vi "JoyToFps.vi"(8 "FpsInput Right":dbl, 9 "FpsInput Left":dbl, 11 "JoystickInput":dbl) -> (0 "Joystick Right":dbl, 1 "Joystick Left":dbl, 3 "Fps":dbl)   [LabVIEW 2020]
doc: "Converts JoystickInput to Fps on top and Fps to joystick on bottom"
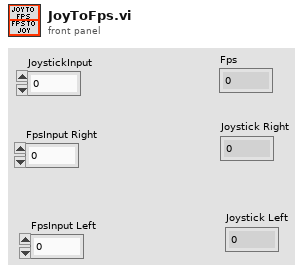
[diagram p1: front panel]
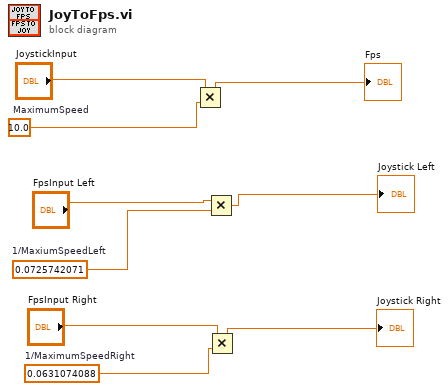
[diagram p0: block diagram]
diagram:
  w1 = 0.0725742071  # 1/MaxiumSpeedLeft
  w5 = 0.0631074088  # 1/MaximumSpeedRight
  w8 = 10.0  # MaximumSpeed
  n1 = Multiply(x="JoystickInput", y=w8) -> (x*y=→"Fps":dbl)
  n2 = Multiply(x="FpsInput Left", y=w1) -> (x*y=→"Joystick Left":dbl)
  n3 = Multiply(x="FpsInput Right", y=w5) -> (x*y=→"Joystick Right":dbl)
